vi "Initialize.vi"(8 "error in (no error)":errorcluster, 11 "subprocess in":refnum<class "Buffered Subprocess.lvclass">) -> (0 "error out":errorcluster, 3 "subprocess out":refnum<class "Buffered Subprocess.lvclass">)   [LabVIEW 2020, in "NI_Subprocess.lvlib" / "Buffered Subprocess.lvclass"]
uses:
  <vilib>/Subprocess/Buffered Subprocess/Buffered Subprocess.lvclass
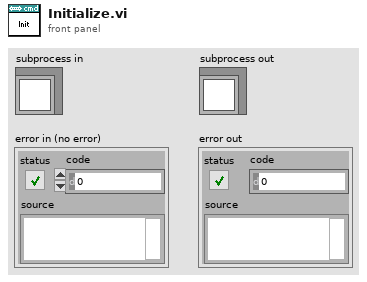
[diagram p1: front panel]
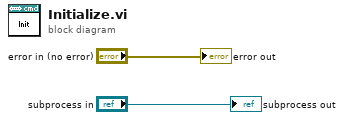
[diagram p0: block diagram]
diagram:
  "error out" <- "error in (no error)"
  "subprocess out" <- "subprocess in"
